vi "16 bit display mapping.vi"(8 "error in (no error)":errorcluster, 10 "16 bit display mapping":cluster{"Low limit":i32, "High limit":i32}, 11 "Image Display":T1) -> (0 "error out":errorcluster, 3 "Image display":T1)   [LabVIEW 2020]
uses:
  Typedefs/Image display ref.ctl
panel:
  in  "Number Of Shifts (255)":i32=255
  in  "Conversion Method (Given Range)":u32(ring)=2 items=["Full Dynamic", "Downshift", "Given Range", "90% Dynamic", "Given Percent Range"]
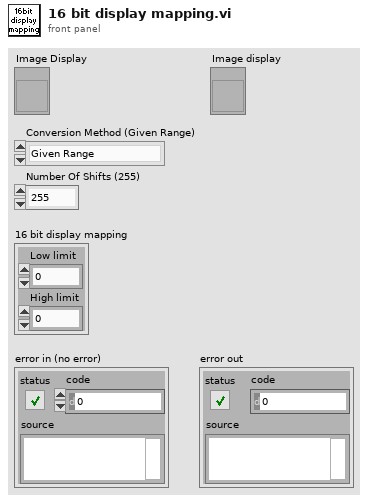
[diagram p1: front panel]
types:
  T1 = typedef "Image display ref.ctl" = refnum<vi>
  T2 = cluster{"Conversion Method":u32, "Minimum Value":i32, "Maximum Value":i32, "Number Of Shifts":i32}
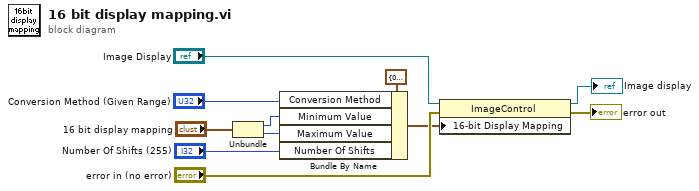
[diagram p0: block diagram]
diagram:
  n1 = Unbundle("16 bit display mapping") -> ("Low limit"=w5:i32, "High limit"=w4:i32)
  n2 = Bundle By Name(cluster=T2 {"Conversion Method"=0, "Minimum Value"=0, "Maximum Value"=0, "Number Of Shifts"=0} ("16-bit Display Mapping:All Elements"), "Conversion Method"="Conversion Method (Given Range)", "Minimum Value"=w5, "Maximum Value"=w4, "Number Of Shifts"="Number Of Shifts (255)") -> (w7:T2)
  n3 = property on="Property Node" class="ImageControl"(reference="Image Display", error in="error in (no error)", "16-bit Display Mapping"=w7) -> (reference out=→"Image display":T1, error out=→"error out":errorcluster)
